vi "Update Label.vi"(8 "error in":errorcluster, 10 "label value":u8 format="%.0o", 11 "32-bit word in":refnum<class "32-bit Word.lvclass">) -> (0 "error out":errorcluster, 3 "32-bit word out":refnum<class "32-bit Word.lvclass">)   [LabVIEW 2020, in "32-bit Word.lvclass"]
uses:
  32-bit Word.lvclass
  C:/Git/Ballard-ARINC429-custom-device/ARINC429/ARINC 429.lvclass
  ARINC 429.lvclass/ARINC 429.ctl
  32-bit Word.lvclass/32-bit Word.ctl
  5c5fc4fb-6106-4363-aed5-f97f5350a028.vi
  Read 32-Bit Word.vi
  Read Label Start Index.vi
  Read Label Size.vi
  Write 32-Bit Word.vi
  5c5fc4fb-6106-4363-aed5-f97f5350a028.vi/a7fcce85-1f75-4572-aeaa-ddfd463a7c5f.vi
  ARINC 429.lvclass
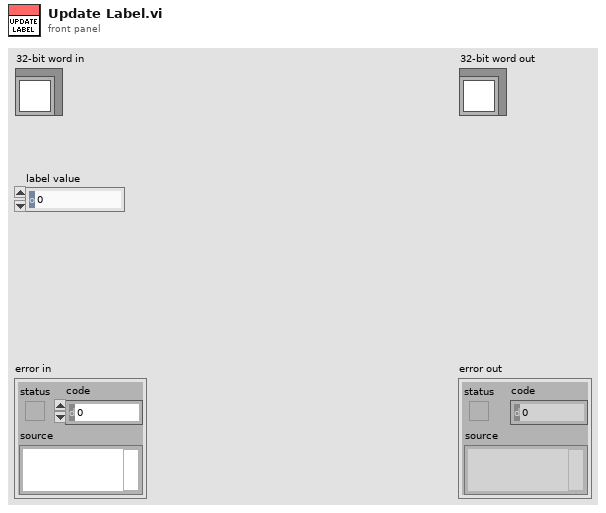
[diagram p1: front panel]
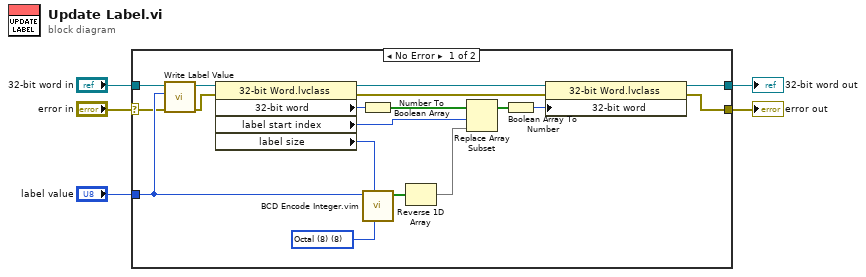
[diagram p0: block diagram]
diagram:
  n1 = case shown="No Error" "error in" {
    selector: "error in" -> [w7 w25]
    tunnel: [w6 w25] -> w4
    tunnel: [w12 w24] -> w2
    tunnel: "32-bit word in" -> [w11 w24]
    tunnel: "label value" -> [w22 _]
    frame No Error {
      w20 = u8 8 items=["Binary (2)"=2, "Octal (8)"=8, "Decimal (10)"=10, "Hexadecimal (16)"=16] ("base")
      n2 = call "Write Label Value.vi"("error in"=w7, "label value"=w22, "ARINC 429 in"=w11) -> ("error out"=w9:errorcluster, "ARINC 429 out"=w23:refnum<class "32-bit Word.lvclass">)  [unwired: 7 in]
      n3 = property class="32-bit Word.lvclass"(reference=w23, error in=w9) -> (reference out=w13:refnum<class "32-bit Word.lvclass">, error out=w8:errorcluster, "32-bit word"=w19:u32, "label start index"=w16:i32, "label size"=w21:i32)
      n4 = Number To Boolean Array(number=w19) -> (Boolean array=w18:bool[])
      n5 = call "BCD Encode Integer.vim"("base"=w20, "data size (bits)"=w21, "integer"=w22) -> ("BCD encoded value"=w17:bool[])  [unwired: 7 in, 1 out]
      n6 = Reverse 1D Array(array=w17) -> (reversed array=w10:bool[])
      n7 = Replace Array Subset(array=w18, new element=w10, index=w16) -> (w15:bool[])
      n8 = Boolean Array To Number(Boolean array=w15) -> (number=w14:u32)
      n9 = property class="32-bit Word.lvclass"(reference=w13, error in=w8, "32-bit word"=w14) -> (reference out=w12:refnum<class "32-bit Word.lvclass">, error out=w6:errorcluster)
    }
    frame Error {
    }
  }
  "error out" <- w4
  "32-bit word out" <- w2
